vi "Write Spell.vi"(8 "error in (no error)":errorcluster, 10 "Spell*":refnum<data-value>, 11 "EnchantedRoom in":refnum<class "EnchantedRoom.lvclass">) -> (0 "error out":errorcluster, 3 "EnchantedRoom out":refnum<class "EnchantedRoom.lvclass">)   [LabVIEW 2016, in "EnchantedRoom.lvclass"]
uses:
  EnchantedRoom.lvclass
  Spell/Spell.lvclass
  EnchantedRoom.lvclass/EnchantedRoom.ctl
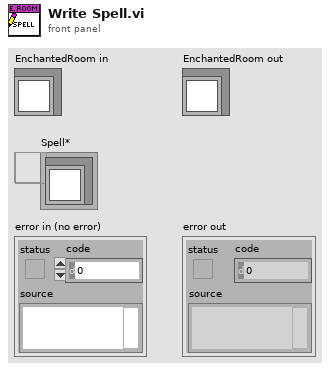
[diagram p1: front panel]
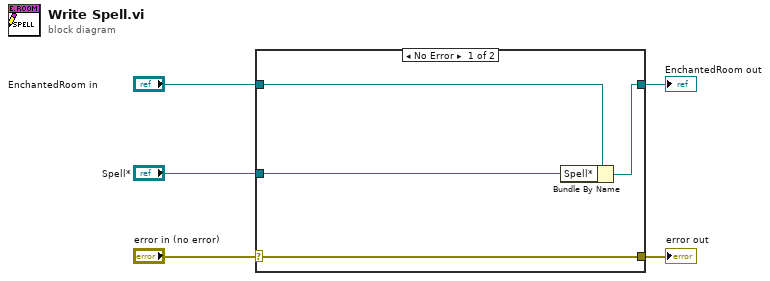
[diagram p0: block diagram]
diagram:
  n1 = case shown="No Error" "error in (no error)" {
    selector: "error in (no error)" -> [w9 w10]
    tunnel: [w9 w10] -> w4
    tunnel: [w7 w11] -> w2
    tunnel: "EnchantedRoom in" -> [w8 w11]
    tunnel: "Spell*" -> [w6 _]
    frame No Error {
      n2 = Bundle By Name(cluster=w8, "Spell*"=w6) -> (w7:refnum<class "EnchantedRoom.lvclass">)
    }
    frame Error {
    }
  }
  "error out" <- w4
  "EnchantedRoom out" <- w2
